vi "TestTakeSingleImage.vi"() -> ()   [LabVIEW 2019]
panel:
  out "size(s)":i32[](array[numeric])
  out "Image Pixels (U16)":u16[][](array[numeric])
  out "Intensity Chart":u16[][](graph)
  out "Image":T1(plugin-control)
  in  "Error In":errorcluster
  out "Error Out":errorcluster
  in  "ExposureTime_us":u32
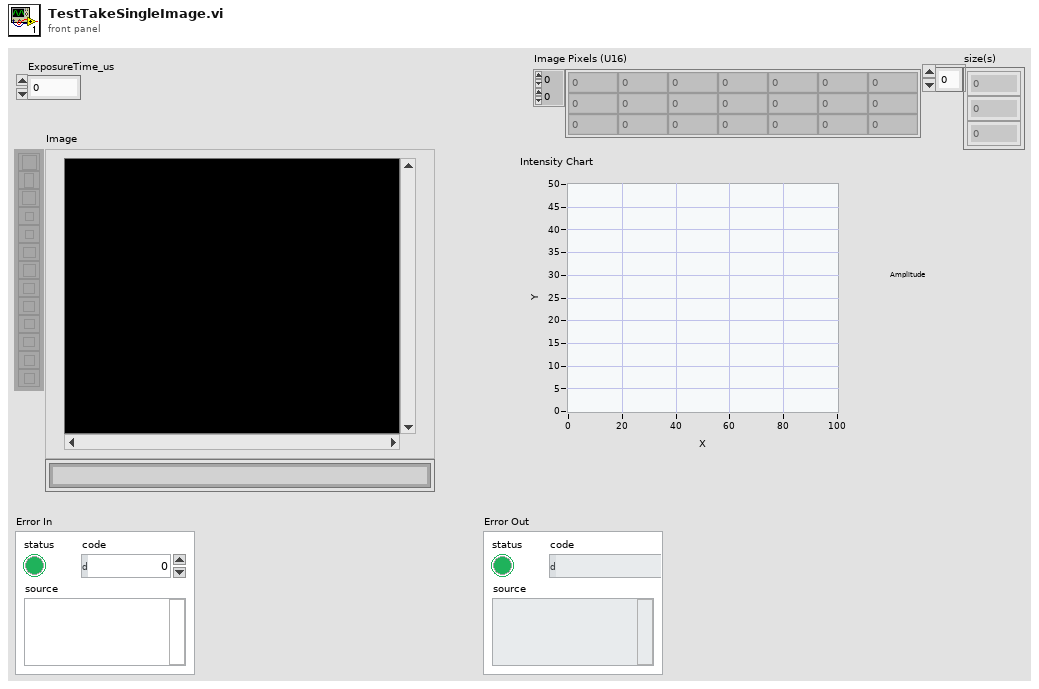
[diagram p1: front panel]
types:
  T1 = typedef "IMAQ Image.ctl" = refnum<image>
  T2 = typedef "Image Type" = u32
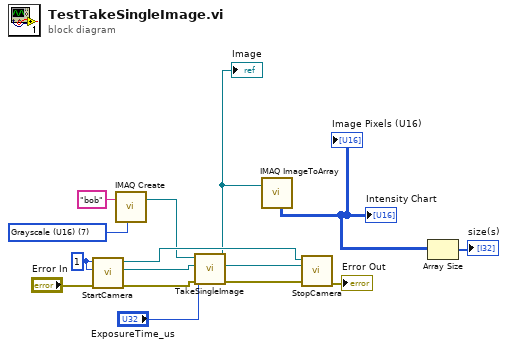
[diagram p0: block diagram]
diagram:
  w1 = T2 7 items=["Grayscale (U8)", "Grayscale (I16)", "Grayscale (SGL)", "Complex (CSG)", "RGB (U32)", "HSL (U32)", "RGB (U64)", "Grayscale (U16)"] ("Image Type")
  w8 = u32 1 ("Gain")
  n1 = call "StartCamera.vi"("Error In"="Error In", "ExposureTime_us"=w8, "Gain"=w8) -> ("Error Out"=w10:errorcluster, "TLCamera reference out"=w13:refnum<k24>, "TLCameraSDK reference out"=w15:refnum<k24>)  [unwired: 6 in]
  n2 = call "IMAQ Create"("Image Name"="bob", "Image Type"=w1) -> ("New Image"=w11:T1)  [unwired: 3 in, 1 out]
  n3 = call "TakeSingleImage.vi"("Image"=w11, "TLCamera reference in"=w13, "ExposureTime_us"="ExposureTime_us", "Error In"=w10) -> ("Image Out"=w4:T1, "TLCamera reference out"=w14:refnum<k24>, "Error Out"=w7:errorcluster)  [unwired: 4 in]
  "Image" <- w4
  n4 = call "IMAQ ImageToArray"("Image"=w4) -> ("Image Pixels (U16)"=w3:u16[][])  [unwired: 3 in, 4 out]
  "Intensity Chart" <- w3
  "Image Pixels (U16)" <- w3
  n5 = call "StopCamera.vi"("Error In"=w7, "TLCamera reference"=w14, "TLCameraSDK reference"=w15) -> ("Error Out"=→"Error Out":errorcluster)  [unwired: 8 in]
  n6 = Array Size(array=w3) -> (size(s)=→"size(s)":i32[])
